vi "DB Open.vi"(8 "error in":errorcluster, 10 "DB":T1={"DataSource Name"="eDCU_LTT", "userID"="root", "password"="edultt"}, 11 "Database in":refnum<class "Database.lvclass">) -> (0 "error out":errorcluster, 3 "Database out":refnum<class "Database.lvclass">)   [LabVIEW 2023, in "HardwareAbstractionLayer_LVOOP.lvlib" / "Database.lvclass"]
doc: "This VI is Database Connection Open"
uses:
  Database.lvclass
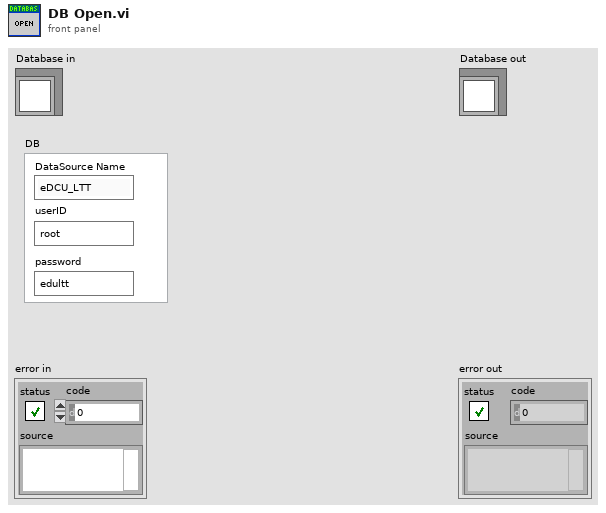
[diagram p1: front panel]
types:
  T1 = cluster{"DataSource Name":string, "userID":string, "password":string}
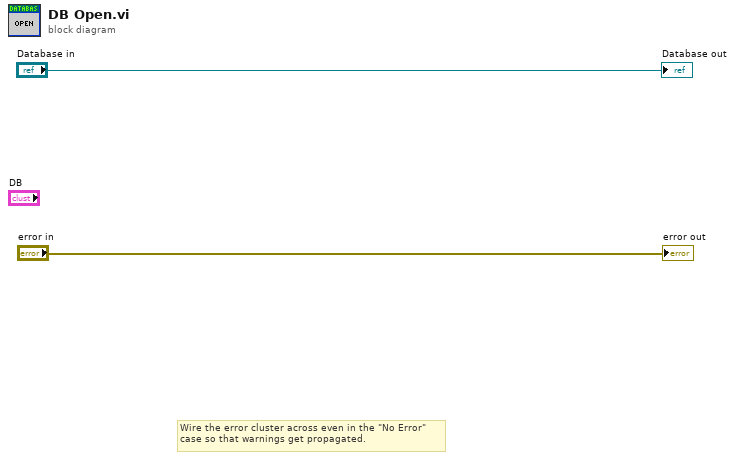
[diagram p0: block diagram]
diagram:
  # "Wire the error cluster across even in the \"No Error\"\ncase so that warnings get propagated."
  "error out" <- "error in"
  "Database out" <- "Database in"
